vi "ReadM2VelocityPID.vi"() -> ()   [LabVIEW 2015]
uses:
  <instrlib>/Ion Motion Roboclaw/Ion Motion Roboclaw.lvlib
panel:
  in  "Address":u8
  out "Kp":u32
  out "Kd":u32
  out "Ki":u32
  out "QPPS":u32
  out "Valid":bool
  out "error out":errorcluster
  in  "COM port":refnum<visa-resource-name>
  in  "baud rate (38400)":u32
  in  "error in (no error)":errorcluster
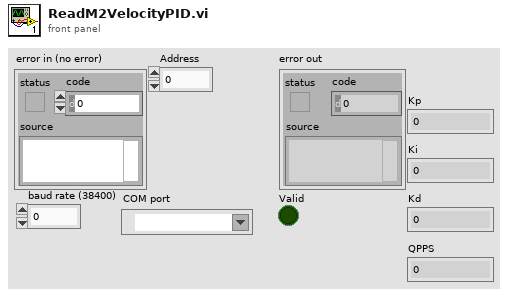
[diagram p1: front panel]
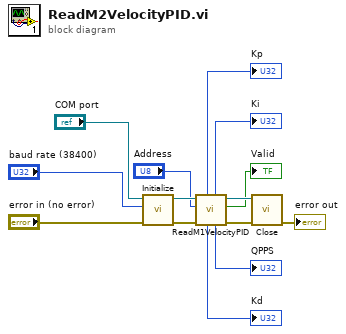
[diagram p0: block diagram]
diagram:
  n1 = call <instrlib>:"Initialize.vi"("error in (no error)"="error in (no error)", "baud rate (38400)"="baud rate (38400)", "COM port"="COM port") -> ("error out"=w13:errorcluster, "VISA resource name out"=w14:refnum<visa-resource-name>)  [unwired: 7 in]
  n2 = call <instrlib>:"ReadM1VelocityPID.vi"("error in (no error)"=w13, "Address"="Address", "VISA Refnum in"=w14) -> ("error out"=w11:errorcluster, "Valid"=→"Valid":bool, "VISA Refnum out"=w12:refnum<visa-resource-name>, "QPPS"=→"QPPS":u32, "Ki"=→"Ki":u32, "Kd"=→"Kd":u32, "Kp"=→"Kp":u32)  [unwired: 2 in]
  n3 = call <instrlib>:"Close.vi"("error in (no error)"=w11, "VISA resource name"=w12) -> ("error out"=→"error out":errorcluster)  [unwired: 9 in]
